vi "start.vi"(8 "error in (no error)":errorcluster, 11 "Model in":refnum<class "Model.lvclass">) -> (0 "error out":errorcluster, 3 "Model out":refnum<class "Model.lvclass">)   [LabVIEW 2013, in "Model.lvclass"]
uses:
  Model.lvclass
  Model.lvclass/Model.ctl
  <userlib>/Common/ILC/ILC/ILC.lvclass/ILC.ctl
  <userlib>/Common/ILC/ILC/ILC.lvclass
  ApplicationElements/SystemController/SystemController.lvclass
  <userlib>/Common/Devices/DistanceGauge/DistanceGauge/DistanceGauge.lvclass
  <userlib>/Common/Devices/ForceSensorCalculator/ForceSensorCalculator/ForceSensorCalculator.lvclass
  ApplicationElements/Thermocouple/Thermocouple.lvclass
  <userlib>/Common/Devices/EncoderReader/EncoderReader/EncoderReader.lvclass
  ApplicationElements/StiffnessMonitor/StiffnessMonitor.lvclass
  <userlib>/Common/Devices/StepperMotor/StepperMotor/StepperMotor.lvclass
  <userlib>/Common/Devices/EncoderConverter/EncoderConverter/EncoderConverter.lvclass
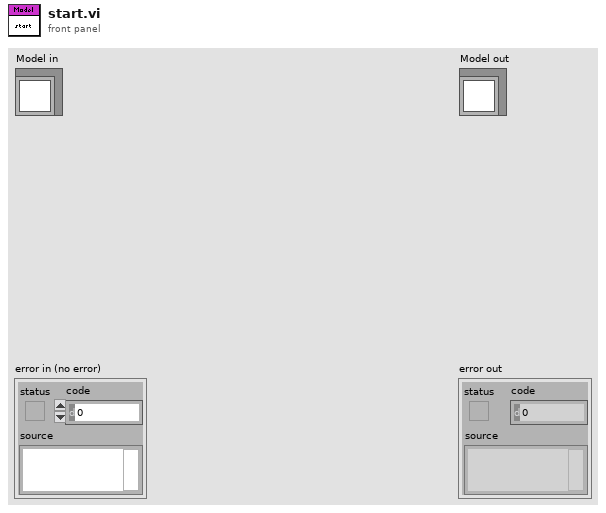
[diagram p1: front panel]
types:
  T1 = typedef "ILCCommon.lvlib/ILCConfiguration.lvlib/ILCADC.ctl" = cluster{"Input Channels":T2, "Scan Rate (Hz) ":T3, "PGA Gain Coefficient":u8, "Reference Voltage Vref":dbl[unit], "Nominal Input Range in Counts":u32, "Preamplifier Gain":u8, "Conversion Settling Cycles":u16}
  T2 = typedef "ILCCommon.lvlib/ILCConfiguration.lvlib/InputChannels.ctl" = enum16{"Channel 0", "3 Channels", "5 Channels"}
  T3 = typedef "ILCCommon.lvlib/ILCConfiguration.lvlib/ScanRate_Hz_MultichannelOptions.ctl" = enum16{"50", "60", "100", "120", "200", "240", "300", "400", "480", "600", "1200", "2400", "4800"}
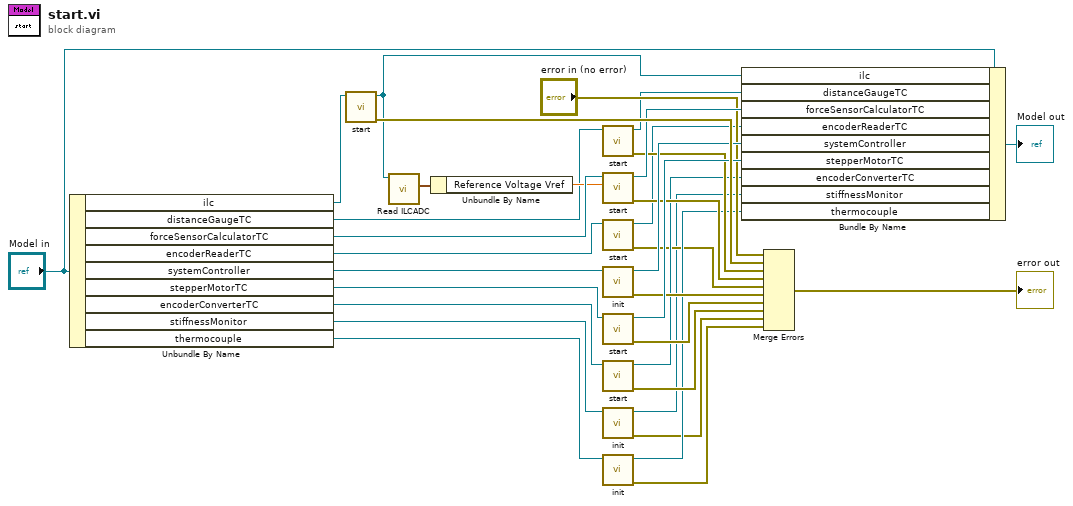
[diagram p0: block diagram]
diagram:
  n1 = Unbundle By Name("Model in") -> ("ilc"=w31:refnum<class "ILC.lvclass">, "distanceGaugeTC"=w10:refnum<class "DistanceGaugeTC.lvclass">, "forceSensorCalculatorTC"=w28:refnum<class "ForceSensorCalculatorTC.lvclass">, "encoderReaderTC"=w5:refnum<class "EncoderReaderTC.lvclass">, "systemController"=w26:refnum<class "SystemController.lvclass">, "stepperMotorTC"=w24:refnum<class "StepperMotorTC.lvclass">, "encoderConverterTC"=w16:refnum<class "EncoderConverterTC.lvclass">, "stiffnessMonitor"=w3:refnum<class "StiffnessMonitor.lvclass">, "thermocouple"=w9:refnum<class "Thermocouple.lvclass">)
  n2 = call <userlib>:"start.vi"("ILC in"=w31) -> ("error out"=w30:errorcluster, "ILC out"=w12:refnum<class "ILC.lvclass">)  [unwired: 9 in]
  n3 = call <userlib>:"Read ILCADC.vi"("ILC in"=w12) -> ("ILC ADC"=w13:T1)  [unwired: 9 in, 1 out]
  n4 = Unbundle By Name(w13) -> ("Reference Voltage Vref"=w11:dbl[unit])
  n5 = call <userlib>:"start.vi"("DistanceGauge in"=w10) -> ("error out"=w17:errorcluster, "DistanceGauge out"=w18:refnum<class "DistanceGaugeTC.lvclass">)  [unwired: 9 in]
  n6 = call <userlib>:"start.vi"("Reference Voltage Vref"=w11, "ForceSensor in"=w28) -> ("error out"=w21:errorcluster, "ForceSensor out"=w27:refnum<class "ForceSensorCalculatorTC.lvclass">)  [unwired: 8 in]
  n7 = call <userlib>:"start.vi"("EncoderReader in"=w5) -> ("error out"=w4:errorcluster, "EncoderReader out"=w6:refnum<class "EncoderReaderTC.lvclass">)  [unwired: 9 in]
  n8 = call "init.vi"("Compensator in"=w26) -> ("error out"=w20:errorcluster, "Compensator out"=w25:refnum<class "SystemController.lvclass">)  [unwired: 9 in]
  n9 = call <userlib>:"start.vi"("StepperMotor in"=w24) -> ("error out"=w19:errorcluster, "StepperMotor out"=w23:refnum<class "StepperMotorTC.lvclass">)  [unwired: 9 in]
  n10 = call <userlib>:"start.vi"("EncoderConverter in"=w16) -> ("error out"=w14:errorcluster, "EncoderConverter out"=w15:refnum<class "EncoderConverterTC.lvclass">)  [unwired: 9 in]
  n11 = call "init.vi"("StiffnessMonitor in"=w3) -> ("error out"=w1:errorcluster, "StiffnessMonitor out"=w2:refnum<class "StiffnessMonitor.lvclass">)  [unwired: 9 in]
  n12 = call "init.vi"("Thermocouple in"=w9) -> ("error out"=w7:errorcluster, "Thermocouple out"=w8:refnum<class "Thermocouple.lvclass">)  [unwired: 9 in]
  n13 = Bundle By Name(cluster="Model in", "ilc"=w12, "distanceGaugeTC"=w18, "forceSensorCalculatorTC"=w27, "encoderReaderTC"=w6, "systemController"=w25, "stepperMotorTC"=w23, "encoderConverterTC"=w15, "stiffnessMonitor"=w2, "thermocouple"=w8) -> (→"Model out":refnum<class "Model.lvclass">)
  n14 = Merge Errors("error in (no error)", w30, w17, w21, w4, w20, w19, w14, w1, w7) -> (→"error out":errorcluster)
